vi "Entire_space_2_Exclude.vi"(1 "Entire Space":T2=[{"Max"=15001.0, "Min"=12000.0}, {"Max"=1000.0, "Min"=-1000.0}, {"Max"=700.0, "Min"=0.0}] {"Min" format="%#.1f"; "Max" format="%#.1f"}) -> (0 "Exculde Array":T1[](array[typedef]) {"Sizes"."Min" format="%#.1f"; "Sizes"."Max" format="%#.1f"})   [LabVIEW 2011]
uses:
  Box_size.ctl
  Exclude_cluster.ctl
  Exclusion_type.ctl
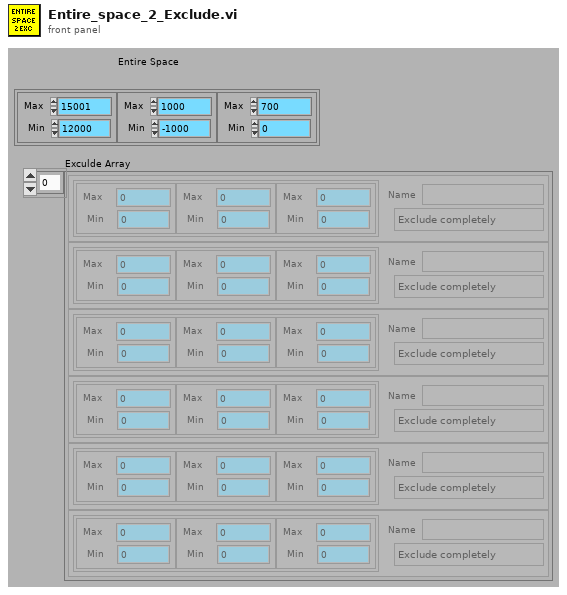
[diagram p1: front panel]
types:
  T1 = typedef "Exclude_cluster.ctl" = cluster{"Sizes":T2, "Name":string, "Exclude Type":T3}
  T2 = typedef "Box_size.ctl" = cluster{"Max":dbl, "Min":dbl}[]
  T3 = typedef "Exclusion_type.ctl" = enum16{"Exclude completely", "Allow only vertical moves"}
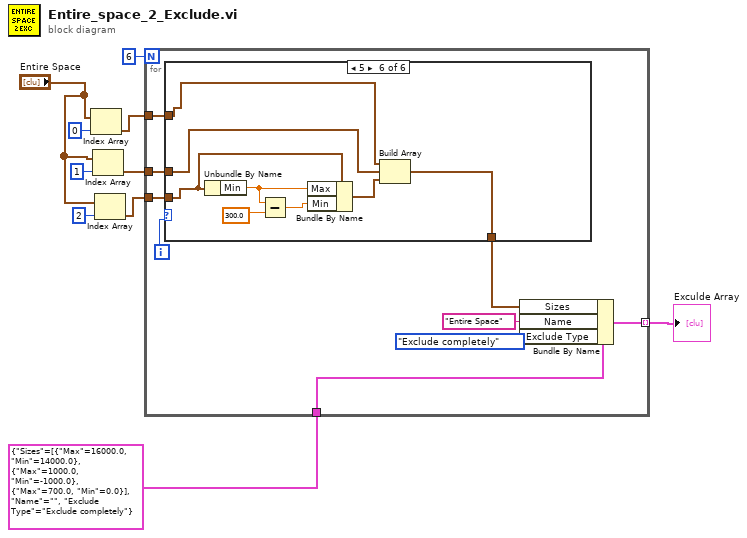
[diagram p0: block diagram]
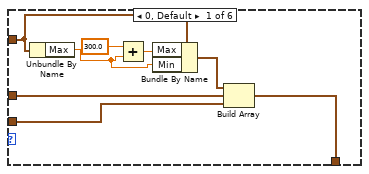
[diagram p2: hidden frame]
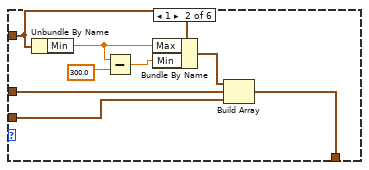
[diagram p3: hidden frame]
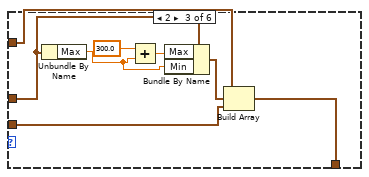
[diagram p4: hidden frame]
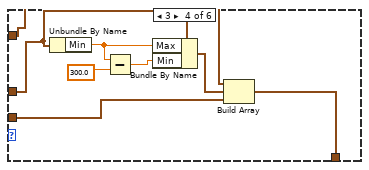
[diagram p5: hidden frame]
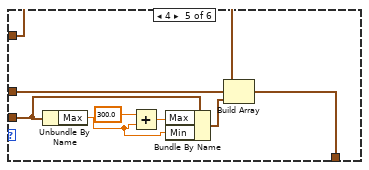
[diagram p6: hidden frame]
diagram:
  n1 = Index Array(array="Entire Space", index=0) -> (element=w2:cluster{"Max":dbl, "Min":dbl})
  n2 = Index Array(array="Entire Space", index=1) -> (element=w4:cluster{"Max":dbl, "Min":dbl})
  n3 = Index Array(array="Entire Space", index=2) -> (element=w3:cluster{"Max":dbl, "Min":dbl})
  n4 = for {
    N: 6 -> [_]
    tunnel: T1 {"Sizes"=[{"Max"=16000.0, "Min"=14000.0}, {"Max"=1000.0, "Min"=-1000.0}, {"Max"=700.0, "Min"=0.0}], "Name"="", "Exclude Type"=enum."Exclude completely"} ("Cluster") -> [w13]
    tunnel: w4 -> [w18]
    tunnel: w3 -> [w17]
    tunnel: w2 -> [w16]
    tunnel: [w11] -> w1 mode=indexing
    i -> [w19]
    n5 = case shown="5" w19 {
      tunnel: w18 -> [w27 w35 w39 w45 w52 w60]
      tunnel: w17 -> [w26 w34 w37 w51 w54 w61]
      tunnel: w16 -> [w25 w33 w36 w44 w55 w63]
      tunnel: [w20 w31 w40 w50 w56 w67] -> w12
      frame 0, Default {
        n6 = Unbundle By Name(w25) -> ("Max"=w21:dbl)
        n7 = Add(x=300.0, y=w21) -> (x+y=w23:dbl)
        n8 = Bundle By Name(cluster=w25, "Max"=w23, "Min"=w21) -> (w24:cluster{"Max":dbl, "Min":dbl})
        n9 = Build Array(w24, w27, w26) -> (w20:cluster{"Max":dbl, "Min":dbl}[])
      }
      frame 1 {
        n10 = Unbundle By Name(w33) -> ("Min"=w28:dbl)
        n11 = Subtract(x=w28, y=300.0 ("x")) -> (x-y=w29:dbl)
        n12 = Bundle By Name(cluster=w33, "Max"=w28, "Min"=w29) -> (w32:cluster{"Max":dbl, "Min":dbl})
        n13 = Build Array(w32, w35, w34) -> (w31:cluster{"Max":dbl, "Min":dbl}[])
      }
      frame 2 {
        n14 = Unbundle By Name(w39) -> ("Max"=w41:dbl)
        n15 = Add(x=300.0, y=w41) -> (x+y=w43:dbl)
        n16 = Bundle By Name(cluster=w39, "Max"=w43, "Min"=w41) -> (w38:cluster{"Max":dbl, "Min":dbl})
        n17 = Build Array(w36, w38, w37) -> (w40:cluster{"Max":dbl, "Min":dbl}[])
      }
      frame 3 {
        n18 = Unbundle By Name(w45) -> ("Min"=w47:dbl)
        n19 = Subtract(x=w47, y=300.0 ("x")) -> (x-y=w48:dbl)
        n20 = Bundle By Name(cluster=w45, "Max"=w47, "Min"=w48) -> (w46:cluster{"Max":dbl, "Min":dbl})
        n21 = Build Array(w44, w46, w51) -> (w50:cluster{"Max":dbl, "Min":dbl}[])
      }
      frame 4 {
        n22 = Unbundle By Name(w54) -> ("Max"=w57:dbl)
        n23 = Add(x=300.0, y=w57) -> (x+y=w59:dbl)
        n24 = Bundle By Name(cluster=w54, "Max"=w59, "Min"=w57) -> (w53:cluster{"Max":dbl, "Min":dbl})
        n25 = Build Array(w55, w52, w53) -> (w56:cluster{"Max":dbl, "Min":dbl}[])
      }
      frame 5 {
        n26 = Unbundle By Name(w61) -> ("Min"=w64:dbl)
        n27 = Subtract(x=w64, y=300.0 ("x")) -> (x-y=w65:dbl)
        n28 = Bundle By Name(cluster=w61, "Max"=w64, "Min"=w65) -> (w62:cluster{"Max":dbl, "Min":dbl})
        n29 = Build Array(w63, w60, w62) -> (w67:cluster{"Max":dbl, "Min":dbl}[])
      }
    }
    n30 = Bundle By Name(cluster=w13, "Sizes"=w12, "Name"="Entire Space", "Exclude Type"=Exclusion_type."Exclude completely") -> (w11:T1)
  }
  "Exculde Array" <- w1
